vi "SetLvClassPath.vi"(0 "reference in":refnum<class "ClassReader.lvclass">, 1 "ClassPath":path, 2 "ClassName":string, 5 "error in (no error)":errorcluster) -> (14 "reference out":refnum<class "ClassReader.lvclass">, 19 "error out":errorcluster)   [LabVIEW 2016, in "ClassReader.lvclass"]
uses:
  <resource>/Framework/Providers/Open_GDS/ClassProviders/Provider_BaseClassInterface/ClassReader_class/ClassReader.lvclass
  <resource>/Framework/Providers/Open_GDS/ClassProviders/Provider_BaseClassInterface/ClassReader_class/ClassReader.lvclass/ClassReader.ctl
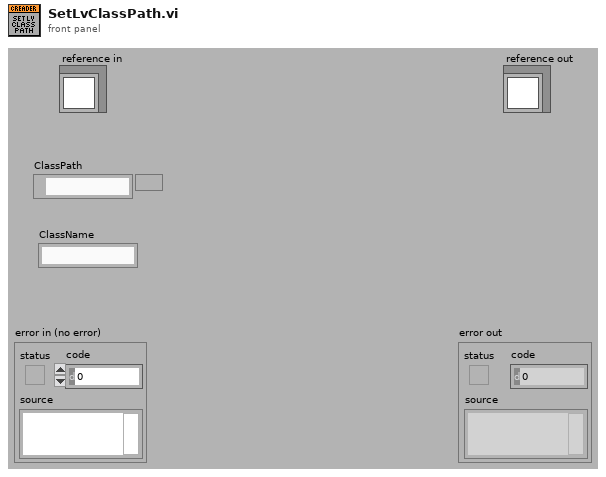
[diagram p1: front panel]
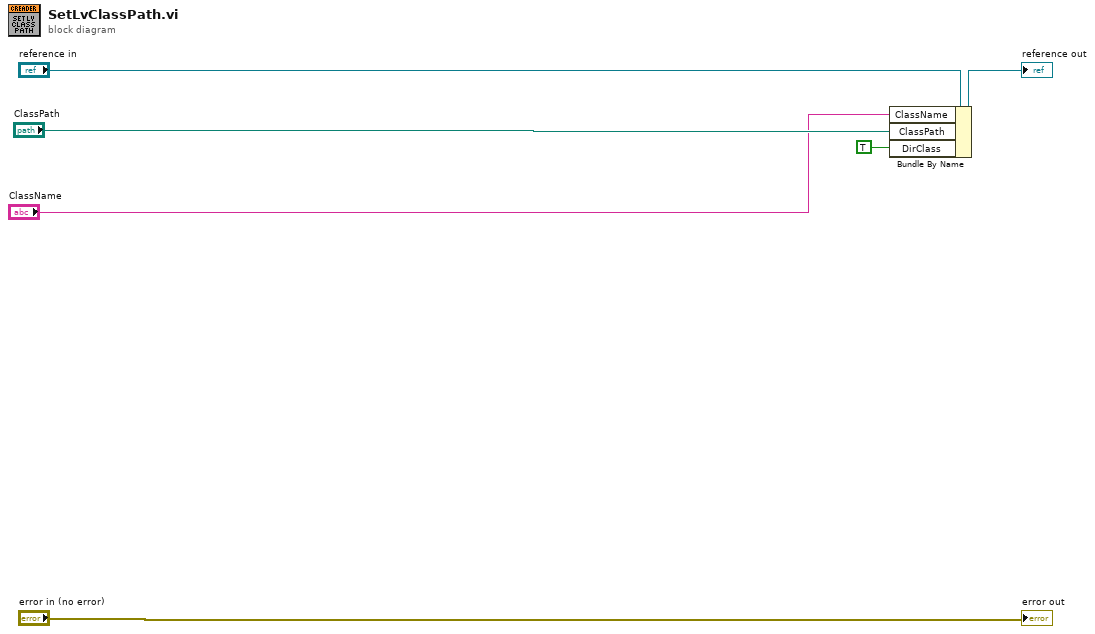
[diagram p0: block diagram]
diagram:
  n1 = Bundle By Name(cluster="reference in", "ClassName"="ClassName", "ClassPath"="ClassPath", "DirClass"=TRUE) -> (→"reference out":refnum<class "ClassReader.lvclass">)
  "error out" <- "error in (no error)"
